vi "GetAllTempSaveNames.vi"() -> ()   [LabVIEW 2012]
uses:
  <vilib>/LVH/i3 JSON/i3-json.lvlib
panel:
  out "element":cluster{"Name":string}
  out "error out":errorcluster
  in  "Config Possible":cluster{"ConfigTemps":cluster{"Name":string}[]}
  in  "String":string
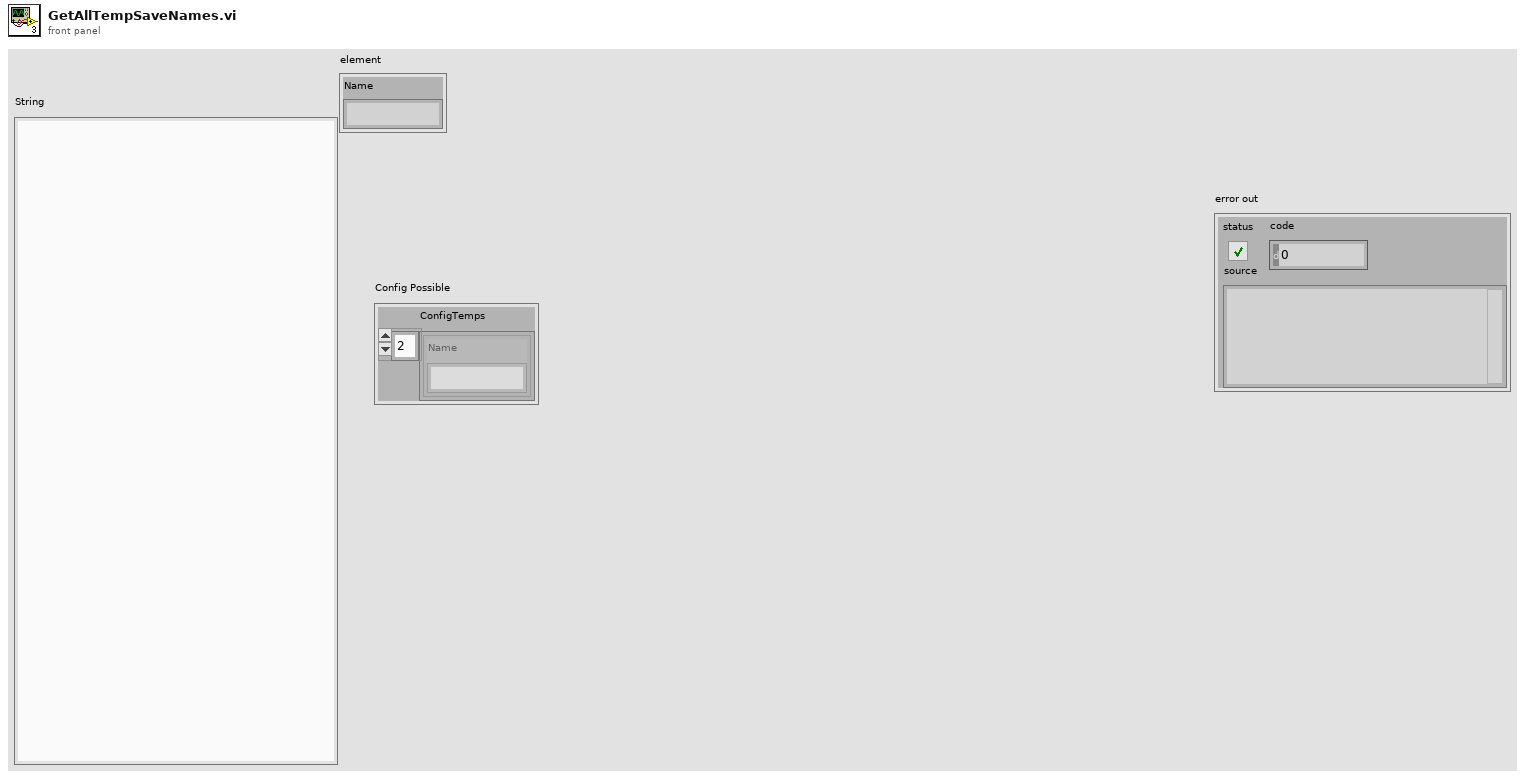
[diagram p1: front panel]
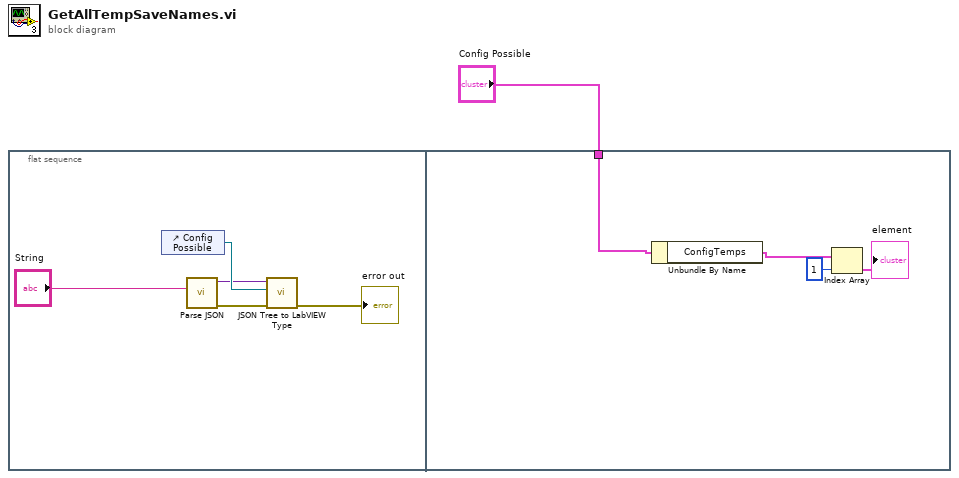
[diagram p0: block diagram]
diagram:
  n1 = flat-sequence {
    tunnel: "Config Possible" -> [w7]
    frame #0 {
      n2 = control-ref of="Config Possible"() -> (w5:refnum<vi>)
      n3 = call <vilib>:"Parse JSON.vi"("JSON String"="String") -> ("error out"=w3:errorcluster, "JSON Tree"=w2:variant)  [unwired: 7 in, 2 out]
      n4 = call <vilib>:"JSON Tree to LabVIEW Type.vi"("error in (no error)"=w3, "Ctl Refnum"=w5, "JSON Tree In"=w2) -> ("error out"=→"error out":errorcluster)  [unwired: 7 in, 1 out]
    }
    frame #1 {
      n5 = Unbundle By Name(w7) -> ("ConfigTemps"=w8:cluster{"Name":string}[])
      n6 = Index Array(array=w8, index=1) -> (element=→"element":cluster{"Name":string})
    }
  }
